vi "meta_createMetaFile.vi"(8 "error in":errorcluster, 11 "file path":path) -> (0 "error out":errorcluster, 3 "meta file":T1)   [LabVIEW 2020, in "NI_ExcelFile.lvlib"]
uses:
  <vilib>/express/express shared/NI_ExcelFile/NI_ExcelFile.lvlib
  <vilib>/express/express shared/NI_ExcelFile/Ctrls/meta_file.ctl
  <vilib>/express/express shared/NI_ExcelFile/Ctrls/meta_Block.ctl
  <vilib>/express/express shared/NI_ExcelFile/Ctrls/meta_BlockType.ctl
  <vilib>/express/express shared/NI_ExcelFile/Ctrls/NITag.ctl
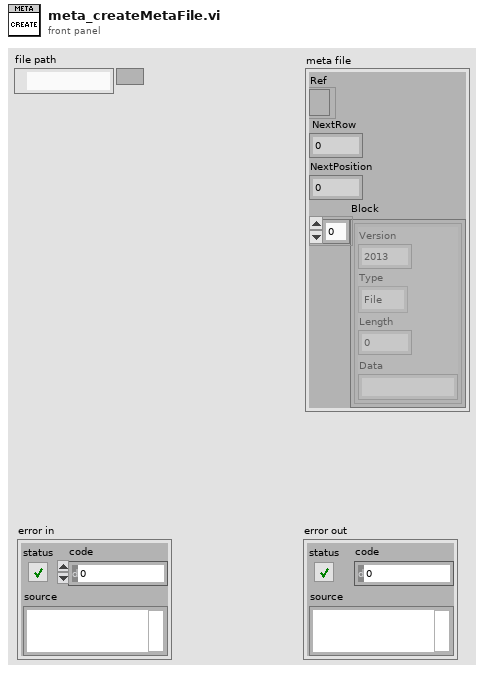
[diagram p1: front panel]
types:
  T1 = typedef "NI_ExcelFile.lvlib/meta_file.ctl" = cluster{"Ref":refnum<file>, "NextRow":i32, "NextPosition":i64, "Block":T2[]}
  T2 = typedef "NI_ExcelFile.lvlib/meta_Block.ctl" = cluster{"Version":u16, "Type":T3, "Length":i32, "Data":string}
  T3 = typedef "NI_ExcelFile.lvlib/meta_BlockType.ctl" = enum16{"NITag", "File", "Column"}
  T4 = enum16{"open", "replace", "create", "open or create", "replace or create", "replace or create with confirmation"}
  T5 = typedef "NI_ExcelFile.lvlib/NITag.ctl" = string
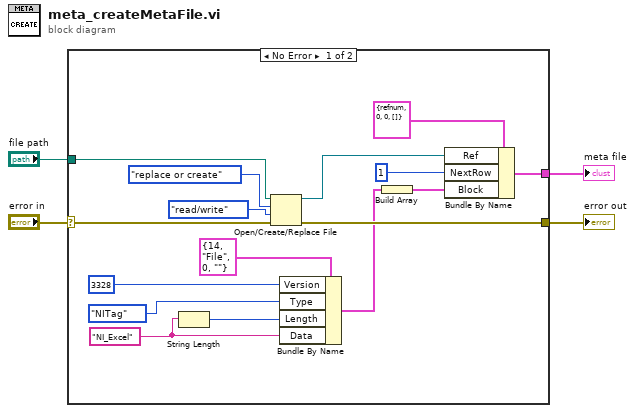
[diagram p0: block diagram]
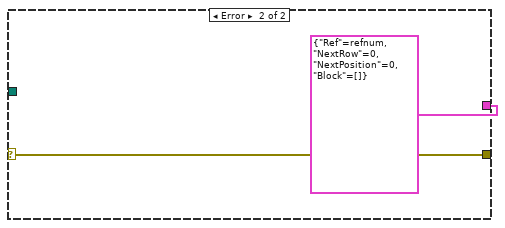
[diagram p2: hidden frame]
diagram:
  n1 = case shown="No Error" "error in" {
    selector: "error in" -> [w15 w21]
    tunnel: "file path" -> [w20 _]
    tunnel: [w17 T1 {"Ref"=refnum, "NextRow"=0, "NextPosition"=0, "Block"=[]} ("meta file")] -> w3
    tunnel: [w6 w21] -> w2
    frame No Error {
      w7 = T5 "NI_Excel" ("NITag")
      n2 = String Length(string=w7) -> (length=w8:i32)
      n3 = Open/Create/Replace File(file path (use dialog)=w20, error in=w15, operation (0:open)=T4."replace or create", access (0:read/write)=enum16{"read/write", "read-only", "write-only"}."read/write") -> (refnum out=w13:refnum<file>, error out=w6:errorcluster)  [unwired: 2 in, 1 out]
      n4 = Bundle By Name(cluster=T2 {"Version"=14, "Type"=enum."File", "Length"=0, "Data"=""} ("Block"), "Version"=u16 3328 ("version"), "Type"=meta_BlockType."NITag" ("type"), "Length"=w8, "Data"=w7) -> (w5:T2)
      n5 = Build Array(w5) -> (w12:T2[])
      n6 = Bundle By Name(cluster=T1 {"Ref"=refnum, "NextRow"=0, "NextPosition"=0, "Block"=[]} ("meta file"), "Ref"=w13, "NextRow"=1, "Block"=w12) -> (w17:T1)
    }
    frame Error {
    }
  }
  "meta file" <- w3
  "error out" <- w2
